vi "sequential on_off - fluigent - v2.vi"() -> ()   [LabVIEW 2018]
doc: "Manually blink and LED attached to a digital output channel of a LINX device by clicking and LED control in LabVIEW."
uses:
  <userlib>/Fluigent/Fluigent MFCS/FluigentMFCS_Full.llb/MFCS_EZ Detect.vi
  <userlib>/Fluigent/Fluigent MFCS/FluigentMFCS_Full.llb/MFCS_EZ Initialization.vi
  <userlib>/Fluigent/Fluigent MFCS/FluigentMFCS_Full.llb/MFCS_EZ Close.vi
panel:
  in  "Delay (ms) (seq 4)":dbl
  in  "Delay_split(ms) (seq 4)":dbl
  in  "Delay_inlet(ms) (seq 4)":dbl
  in  "Alpha_split (def: 5) (seq 4)":u8=5
  in  "split_ch (seq 4)":u8=1
  in  "split_low (seq 4)":dbl
  in  "split_high (seq 4)":dbl
  in  "Alpha_inlet (def: 5) (seq 4)":u8=5
  in  "inlet_ch (seq 4)":u8=1
  in  "inlet_low (seq 4)":dbl
  in  "inlet_high (seq 4)":dbl
  in  "Delay (ms) (seq 3)":dbl
  in  "Delay_split(ms) (seq 3)":dbl
  in  "Delay_inlet(ms) (seq 3)":dbl
  in  "Alpha_split (def: 5) (seq 3)":u8=5
  in  "split_ch (seq 3)":u8=1
  in  "split_low (seq 3)":dbl
  in  "split_high (seq 3)":dbl
  in  "Alpha_inlet (def: 5) (seq 3)":u8=5
  in  "inlet_ch (seq 3)":u8=1
  in  "inlet_low (seq 3)":dbl
  in  "inlet_high (seq 3)":dbl
  in  "Delay (ms) (seq 2)":dbl
  in  "Delay_split(ms) (seq 2)":dbl
  in  "Delay_inlet(ms) (seq 2)":dbl
  in  "Alpha_split (def: 5) (seq 2)":u8=5
  in  "split_ch (seq 2)":u8=1
  in  "split_low (seq 2)":dbl
  in  "split_high (seq 2)":dbl
  in  "Alpha_inlet (def: 5) (seq 2)":u8=5
  in  "inlet_ch (seq 2)":u8=1
  in  "inlet_low (seq 2)":dbl
  in  "inlet_high (seq 2)":dbl
  in  "seq_3_delay":u32
  in  "seq_2_delay":u32
  in  "seq_1_delay":u32
  in  "Delay (ms) (seq 1)":dbl
  in  "Delay_split(ms) (seq 1)":dbl
  in  "Delay_inlet(ms) (seq 1)":dbl
  in  "Alpha_split (def: 5) (seq 1)":u8=5
  in  "split_ch (seq 1)":u8=1
  in  "split_low (seq 1)":dbl
  in  "split_high (seq 1)":dbl
  in  "Alpha_inlet (def: 5) (seq 1)":u8=5
  in  "inlet_ch (seq 1)":u8=1
  in  "inlet_low (seq 1)":dbl
  in  "inlet_high (seq 1)":dbl
  in  "Start Sequence":bool
  in  "stop":bool
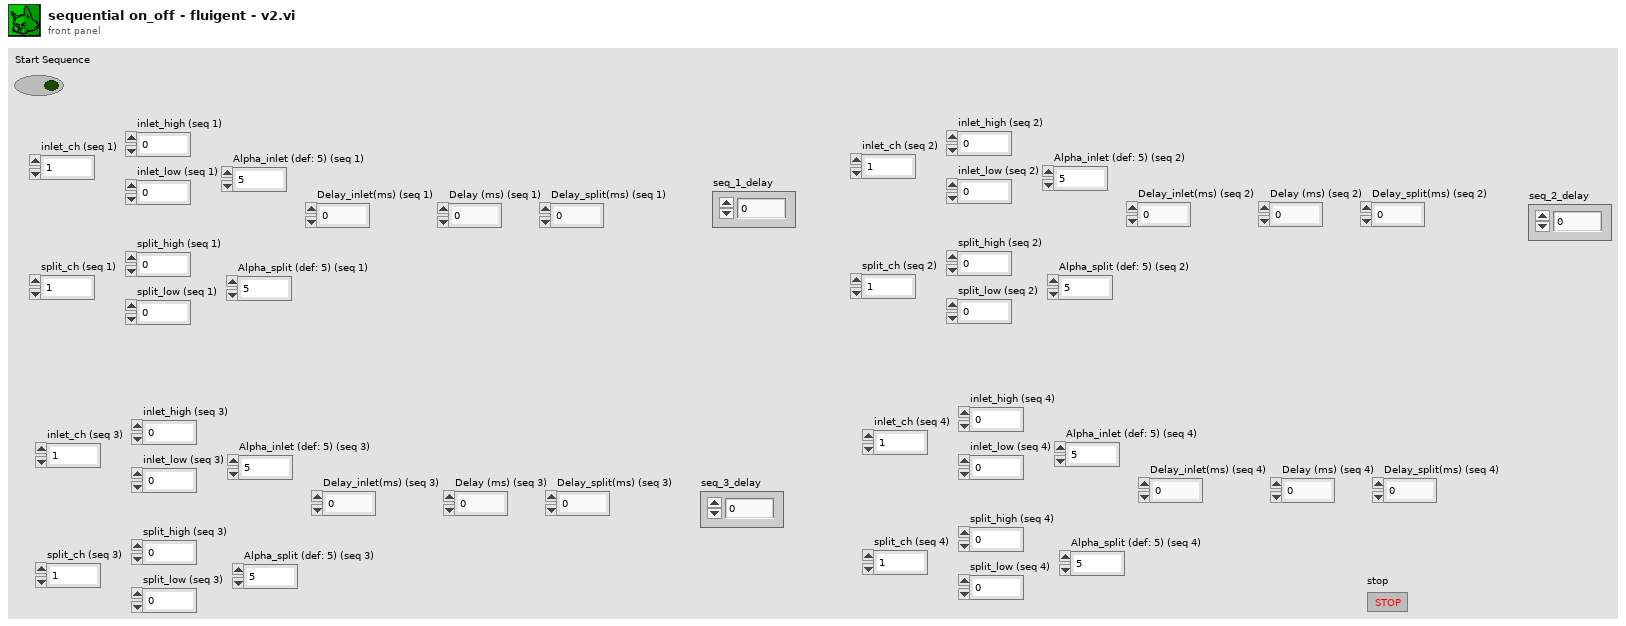
[diagram p1: front panel]
types:
  T1 = typedef "_EZmfcsSN.ctl" = u16
  T2 = typedef "_mfcs_EZ_handle.ctl" = u64
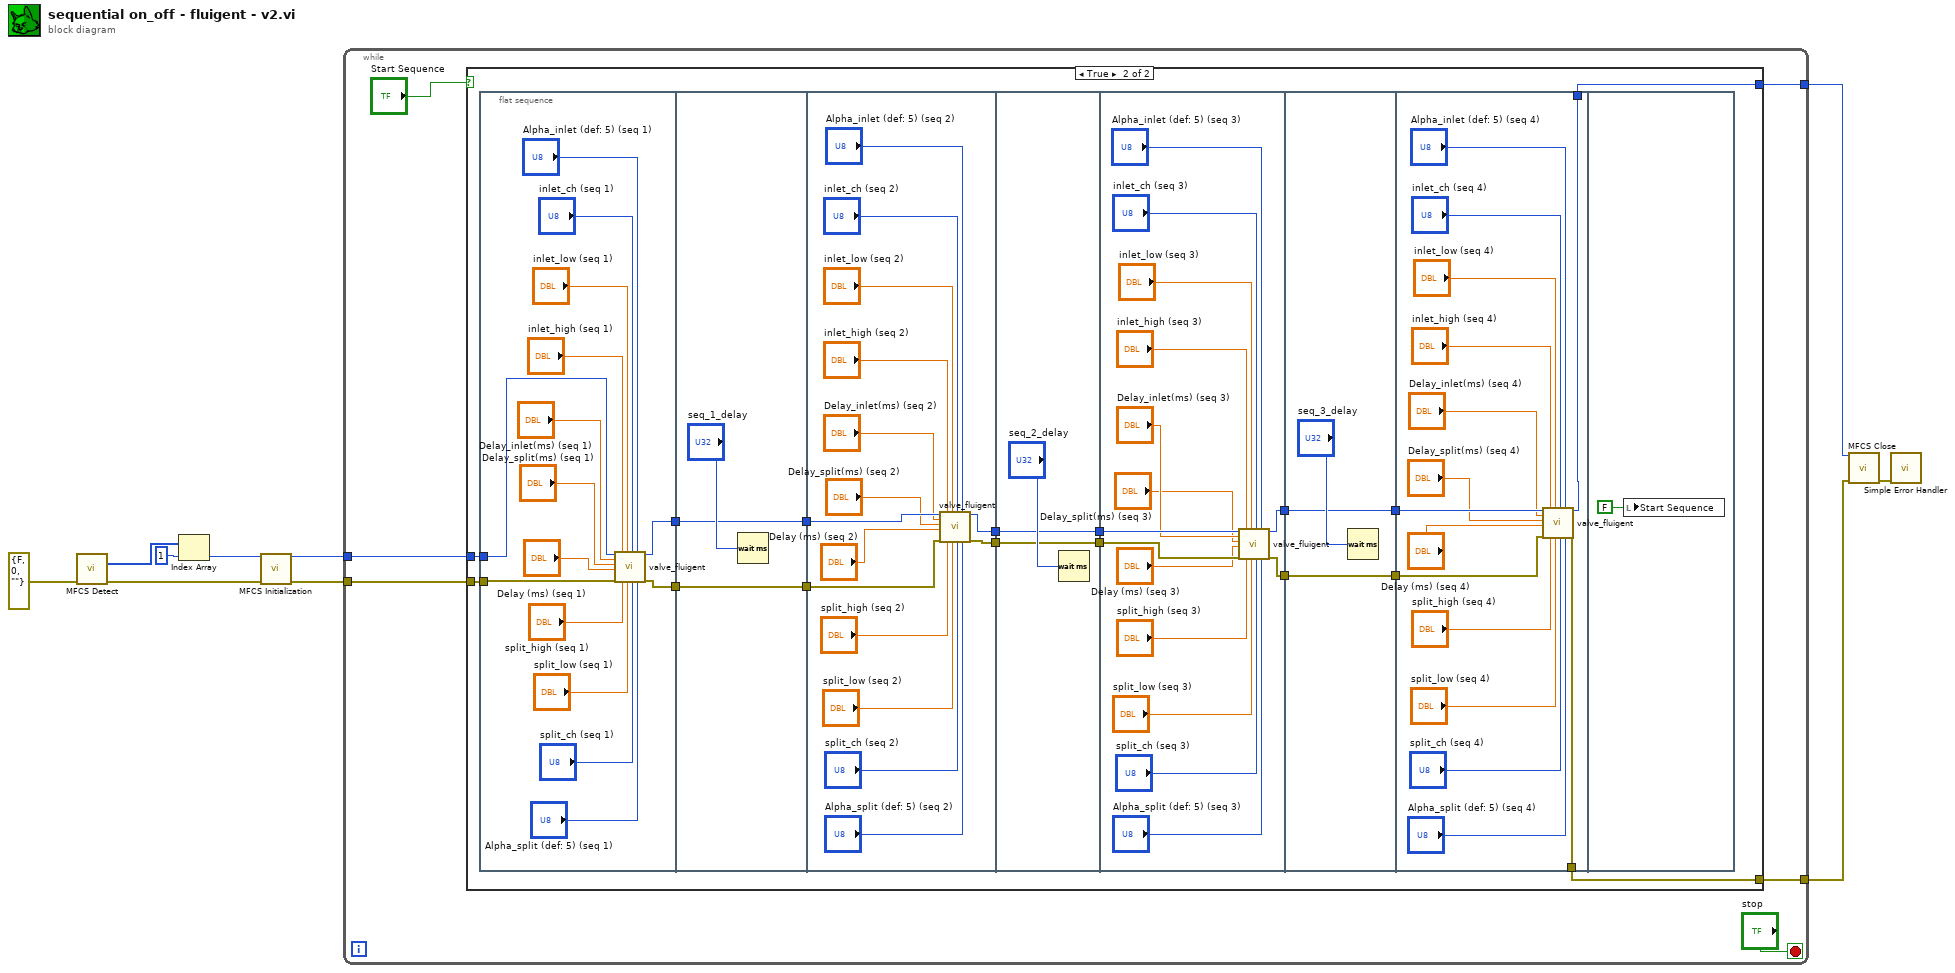
[diagram p0: block diagram]
diagram:
  n1 = call-poly <userlib>:"MFCS Detect.vi"("error in (no error)"=errorcluster {"status"=FALSE, "code"=0, "source"=""}) -> ("[SN MFCS_EZ]"=w9:T1[], "error out"=w8:errorcluster)  [unwired: 13 in]
  n2 = Index Array(array=w9, index=1) -> (element=w7:T1)
  n3 = call-poly <userlib>:"MFCS Initialization.vi"("SN MFCS_EZ"=w7, "error in (no error)"=w8) -> ("MFCS_EZ_out"=w5:T2, "error out"=w6:errorcluster)  [unwired: 10 in, 2 out]
  n4 = while {
    tunnel: w6 -> [w13]
    tunnel: w5 -> [w14]
    tunnel: [w12] -> w2
    tunnel: [w11] -> w1
    stop <- "stop" stop-if-true
    n5 = case shown="True" "Start Sequence" {
      tunnel: w14 -> [w17 w34]
      tunnel: w13 -> [w18 w33]
      tunnel: [w18 w20] -> w12
      tunnel: [w17 w19] -> w11
      frame False {
      }
      frame True {
        n6 = flat-sequence {
          tunnel: w34 -> [w49]
          tunnel: w33 -> [w48]
          tunnel: [w36] -> w31
          tunnel: [w35] -> w30
          tunnel: [w51] -> w32
          tunnel: w31 -> [w51]
          tunnel: w30 -> [w50]
          tunnel: [w50] -> w29
          tunnel: w32 -> [w63]
          tunnel: w29 -> [w55]
          tunnel: [w54] -> w27
          tunnel: [w53] -> w26
          tunnel: [w69] -> w28
          tunnel: w27 -> [w69]
          tunnel: w26 -> [w68]
          tunnel: [w68] -> w25
          tunnel: w28 -> [w81]
          tunnel: w25 -> [w80]
          tunnel: [w72] -> w23
          tunnel: [w71] -> w21
          tunnel: [w87] -> w24
          tunnel: w23 -> [w87]
          tunnel: [w86] -> w22
          tunnel: w21 -> [w86]
          tunnel: w24 -> [w103]
          tunnel: w22 -> [w102]
          tunnel: [w101] -> w20
          tunnel: [w100] -> w19
          frame #0 {
            n7 = call "valve_fluigent.vi"("MFCS_EZ_"=w49, "Delay_inlet(ms)"="Delay_inlet(ms) (seq 1)", "Delay_split(ms)"="Delay_split(ms) (seq 1)", "Delay (ms)"="Delay (ms) (seq 1)", "error in (no error)"=w48, "inlet_high"="inlet_high (seq 1)", "split_high"="split_high (seq 1)", "inlet_low"="inlet_low (seq 1)", "split_low"="split_low (seq 1)", "inlet_ch"="inlet_ch (seq 1)", "split_ch"="split_ch (seq 1)", "Alpha_inlet (def: 5)"="Alpha_inlet (def: 5) (seq 1)", "Alpha_split (def: 5)"="Alpha_split (def: 5) (seq 1)") -> ("MFCS_EZ out"=w36:T2, "error out"=w35:errorcluster)  [unwired: 5 in]
          }
          frame #1 {
            n8 = Wait (ms)(milliseconds to wait="seq_1_delay") -> ()  [unwired: 1 out]
          }
          frame #2 {
            n9 = call "valve_fluigent.vi"("MFCS_EZ_"=w63, "Delay_inlet(ms)"="Delay_inlet(ms) (seq 2)", "Delay_split(ms)"="Delay_split(ms) (seq 2)", "Delay (ms)"="Delay (ms) (seq 2)", "error in (no error)"=w55, "inlet_high"="inlet_high (seq 2)", "split_high"="split_high (seq 2)", "inlet_low"="inlet_low (seq 2)", "split_low"="split_low (seq 2)", "inlet_ch"="inlet_ch (seq 2)", "split_ch"="split_ch (seq 2)", "Alpha_inlet (def: 5)"="Alpha_inlet (def: 5) (seq 2)", "Alpha_split (def: 5)"="Alpha_split (def: 5) (seq 2)") -> ("MFCS_EZ out"=w54:T2, "error out"=w53:errorcluster)  [unwired: 5 in]
          }
          frame #3 {
            n10 = Wait (ms)(milliseconds to wait="seq_2_delay") -> ()  [unwired: 1 out]
          }
          frame #4 {
            n11 = call "valve_fluigent.vi"("MFCS_EZ_"=w81, "Delay_inlet(ms)"="Delay_inlet(ms) (seq 3)", "Delay_split(ms)"="Delay_split(ms) (seq 3)", "Delay (ms)"="Delay (ms) (seq 3)", "error in (no error)"=w80, "inlet_high"="inlet_high (seq 3)", "split_high"="split_high (seq 3)", "inlet_low"="inlet_low (seq 3)", "split_low"="split_low (seq 3)", "inlet_ch"="inlet_ch (seq 3)", "split_ch"="split_ch (seq 3)", "Alpha_inlet (def: 5)"="Alpha_inlet (def: 5) (seq 3)", "Alpha_split (def: 5)"="Alpha_split (def: 5) (seq 3)") -> ("MFCS_EZ out"=w72:T2, "error out"=w71:errorcluster)  [unwired: 5 in]
          }
          frame #5 {
            n12 = Wait (ms)(milliseconds to wait="seq_3_delay") -> ()  [unwired: 1 out]
          }
          frame #6 {
            n13 = call "valve_fluigent.vi"("MFCS_EZ_"=w103, "Delay_inlet(ms)"="Delay_inlet(ms) (seq 4)", "Delay_split(ms)"="Delay_split(ms) (seq 4)", "Delay (ms)"="Delay (ms) (seq 4)", "error in (no error)"=w102, "inlet_high"="inlet_high (seq 4)", "split_high"="split_high (seq 4)", "inlet_low"="inlet_low (seq 4)", "split_low"="split_low (seq 4)", "inlet_ch"="inlet_ch (seq 4)", "split_ch"="split_ch (seq 4)", "Alpha_inlet (def: 5)"="Alpha_inlet (def: 5) (seq 4)", "Alpha_split (def: 5)"="Alpha_split (def: 5) (seq 4)") -> ("MFCS_EZ out"=w100:T2, "error out"=w101:errorcluster)  [unwired: 5 in]
          }
          frame #7 {
            n14 = local write "Start Sequence"(FALSE) -> ()
          }
        }
      }
    }
  }
  n15 = call-poly <userlib>:"MFCS Close.vi"("MFCS_EZ"=w1, "error in (no error)"=w2) -> ("error out"=w4:errorcluster)  [unwired: 13 in]
  n16 = call <vilib>:"Simple Error Handler.vi"("error in (no error)"=w4) -> ()  [unwired: 4 in, 5 out]
